vi "Wake up Helper Loop.vi"(8 "error in":errorcluster, 10 "HL Arguments":T1, 11 "Local Events":T2) -> (0 "error out":errorcluster)   [LabVIEW 2020, in "TDS1002 Oscilloscope.lvlib" / "Local Events.lvlib"]
doc: "____\nPantherLAB Templates 1.0.0.5\nCopyright (c) 2022, PantherLAB\n\n<b>Note:</b> This VI was modified by the <b>Validate DQMH Module</b> tool to be shared clone reentrant."
uses:
  Local Events.lvlib
  Local Events--cluster.ctl
  Helper loop arguments--cluster.ctl
  TDS1002 Oscilloscope.lvlib
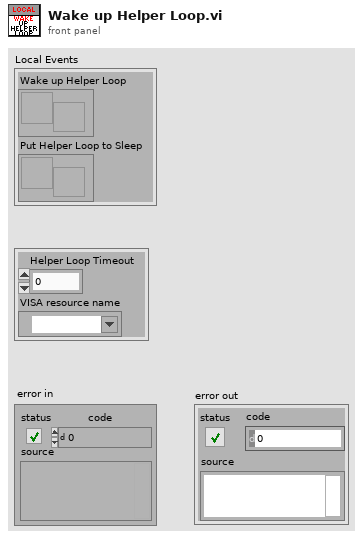
[diagram p1: front panel]
types:
  T1 = typedef "TDS1002 Oscilloscope.lvlib/Helper loop arguments--cluster.ctl" = cluster{"Helper Loop Timeout":i32, "VISA resource name":refnum<visa-resource-name>}
  T2 = typedef "TDS1002 Oscilloscope.lvlib/Local Events.lvlib/Local Events--cluster.ctl" = cluster{"Wake up Helper Loop":refnum<user-event>, "Put Helper Loop to Sleep":refnum<user-event>}
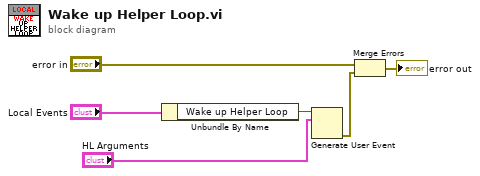
[diagram p0: block diagram]
diagram:
  n1 = Unbundle By Name("Local Events") -> ("Wake up Helper Loop"=w2:refnum<user-event>)
  n2 = Generate User Event(user event=w2, event data cluster="HL Arguments") -> (error out=w5:errorcluster)  [unwired: 2 in, 1 out]
  n3 = Merge Errors("error in", w5) -> (→"error out":errorcluster)
